vi "Save PNG Image (Memory).vi"(8 "error in (no error)":errorcluster, 9 "Compression (6)":i32=6, 10 "Image":T1) -> (0 "error out":errorcluster, 3 "Encoded Image":u8[](array[numeric]))   [LabVIEW 2020, in "G-Image.lvlib"]
doc: "Saves an image in PNG format to disk or memory.\n\nThe <b>Compression</b> input is from 0 to 10, with 0 being no compression and 10 being maximum compression. Values outside this range will be coerced in range."
uses:
  G-Image.lvlib
  <vilib>/picture/picture.llb/imagedata.ctl
  Controls/Image Save Format.ctl
  23d07dd8-0246-46c8-8885-479f1b0fb2b3.vi
  Private/Result To Error.vi
  Private/Get Image Data.vi
  Private/ARGB To RGBA.vi
  Private/Depth To Number Channels.vi
  Image Processing/Indexed Color To True Color Image.vi
  <vilib>/Utility/error.llb/Error Cluster From Error Code.vi
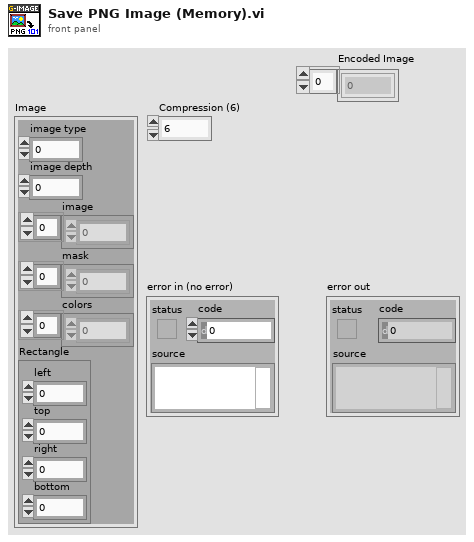
[diagram p1: front panel]
types:
  T1 = typedef "imagedata.ctl" = cluster{"image type":i32, "image depth":i32, "image":u8[], "mask":u8[], "colors":u32[], "Rectangle":cluster{"left":i16, "top":i16, "right":i16, "bottom":i16}}
  T2 = typedef "G-Image.lvlib/Image Save Format.ctl" = enum16{"png", "jpg", "bmp", "gif", "tga", "qoi"}
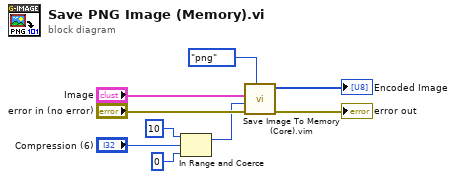
[diagram p0: block diagram]
diagram:
  n1 = In Range and Coerce(upper limit=10, x="Compression (6)", lower limit=0) -> (coerced(x)=w1:i32)  [unwired: 1 out]
  n2 = call "Save Image To Memory (Core).vim"("Save Format"=Image_Save_Format."png", "error in (no error)"="error in (no error)", "Option"=w1, "Image"="Image") -> ("error out"=→"error out":errorcluster, "Encoded Image"=→"Encoded Image":u8[])  [unwired: 6 in]
